vi "setFPGA.vi"(10 "FPGA":refnum<class "FPGA.lvclass">, 11 "ModbusIRQ in":refnum<class "ModbusIRQ.lvclass">) -> (3 "ModbusIRQ out":refnum<class "ModbusIRQ.lvclass">)   [LabVIEW 2016, in "ModbusIRQ.lvclass"]
uses:
  ModbusIRQ.lvclass
  FPGA/FPGA.lvclass
  ModbusIRQ.lvclass/ModbusIRQ.ctl
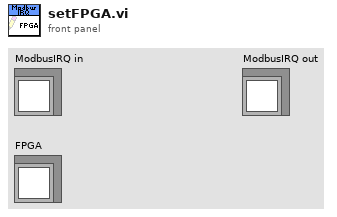
[diagram p1: front panel]
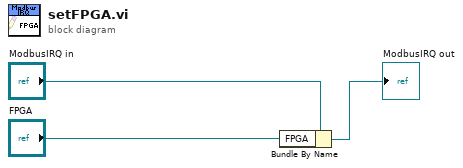
[diagram p0: block diagram]
diagram:
  n1 = Bundle By Name(cluster="ModbusIRQ in", "FPGA"="FPGA") -> (→"ModbusIRQ out":refnum<class "ModbusIRQ.lvclass">)
